vi "GD_Errors_Message.vi"(8 "Errors woanders in":bool, 11 "Sprachliste":string[][](array[string])) -> (0 "Errors":bool, 2 "ErrorMessage PDF":string, 3 "ErrorMessages LogFile":string)   [LabVIEW 2020, in "Linearisierung v2.lvlib" / "SpanEinstellungen.lvlib"]
uses:
  SpanEinstellungen.lvlib
  Aktion FGV Stoerungen sammeln und auswerten.ctl
  Linearisierung v2.lvlib
  Sprachverwaltung/Sprachverwaltung.lvlib
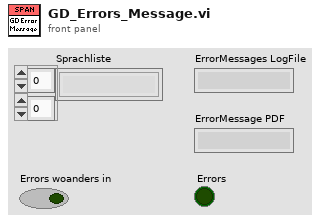
[diagram p1: front panel]
types:
  T1 = typedef "Linearisierung v2.lvlib/Aktion FGV Stoerungen sammeln und auswerten.ctl" = enum16{"init", "lesen", "error", "prüfen", "reset error", "abbrechen", "fortsetzen", "neustart", "Bedientasten reset"}
  T2 = typedef "Linearisierung v2.lvlib/LIN ErrorCluster.ctl" = cluster{"Störung Kommunikation":bool, "Pressure carrier gas":bool, "Pressure diluted gas":bool, "Outlet Pressure":bool, "SNOX before SAIR":bool, "Störung Gasteiler":bool}
  T3 = cluster{"Label.Text":string, "Störung Kommunikation":bool}[]
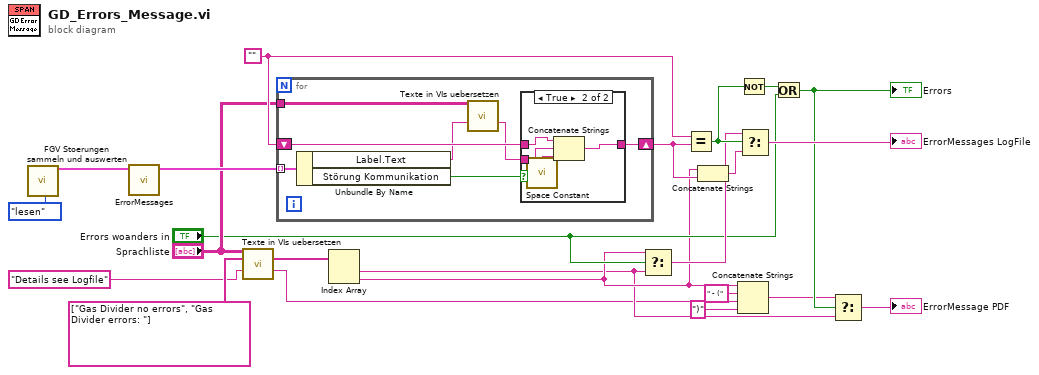
[diagram p0: block diagram]
diagram:
  w19 = ""
  n1 = call "FGV Stoerungen sammeln und auswerten.vi"("Aktion"=Aktion_FGV_Stoerungen_sammeln_und_auswerten."lesen") -> ("Errors"=w17:T2)  [unwired: 12 in, 6 out]
  n2 = call "ErrorMessages.vi"("Errors"=w17) -> ("Error Array"=w18:T3)  [unwired: 9 in, 1 out]
  n3 = call "Texte in VIs uebersetzen.vi"("Sprachliste"="Sprachliste", "String-Array zum Übersetzen"=string[] ["Gas Divider no errors", "Gas Divider errors: "] ("t"), "String zum Übersetzen"="Details see Logfile") -> ("String-Array zum Übersetzen"=w14:string[], "String zum Übersetzen"=w4:string)  [unwired: 8 in, 3 out]
  n4 = for {
    tunnel: w18 -> [w30] mode=indexing
    shift-right: [w28] -> w21
    shift-left: w19 -> [w27]
    tunnel: "Sprachliste" -> [w26]
    n5 = Unbundle By Name(w30) -> ("Label.Text"=w25:string, "Störung Kommunikation"=w29:bool)
    n6 = call "Texte in VIs uebersetzen.vi"("Sprachliste"=w26, "String zum Übersetzen"=w25) -> ("String zum Übersetzen"=w24:string)  [unwired: 9 in, 4 out]
    n7 = case shown="True" w29 {
      tunnel: w24 -> [_ w35]
      tunnel: [w31 w34] -> w28
      tunnel: w27 -> [w31 w32]
      frame False {
      }
      frame True {
        n8 = call <vilib>:"Space Constant.vi"() -> ("String"=w33:string)
        n9 = Concatenate Strings(w32, w35, w33) -> (w34:string)
      }
    }
  }
  n10 = Index Array(array=w14) -> (element #1=w7:string, element #2=w8:string)  [unwired: 2 in]
  n11 = Select(t=w8, s="Errors woanders in", f=w7) -> (s? t:f=w11:string)
  n12 = Equal?(x=w19, y=w21) -> (x = y?=w20:bool)
  n13 = Concatenate Strings(w8, w21) -> (w23:string)
  n14 = Concatenate Strings(w8, " - (" ("String"), w4, ")" ("String")) -> (w6:string)
  n15 = Not(x=w20) -> (.not. x?=w13:bool)
  n16 = Select(t=w11, s=w20, f=w23) -> (s? t:f=→"ErrorMessages LogFile":string)
  n17 = Or(x=w13, y="Errors woanders in") -> (x .or. y?=w9:bool)
  "Errors" <- w9
  n18 = Select(t=w6, s=w9, f=w7) -> (s? t:f=→"ErrorMessage PDF":string)
